vi "Launcher.vi"   [LabVIEW 2019]
uses:
  My First Actor.lvclass
  C:/Program Files (x86)/National Instruments/LabVIEW 2019/vi.lib/ActorFramework/Actor/Actor.lvclass
  My First Actor Messages/PopUp Msg/PopUp Msg.lvclass/PopUp Msg.ctl
  <vilib>/ActorFramework/Message Enqueuer/Message Enqueuer.lvclass/Message Enqueuer.ctl
  My First Actor Messages/PopUp2 Msg/PopUp2 Msg.lvclass/PopUp2 Msg.ctl
  <vilib>/ActorFramework/Message Enqueuer/Enqueue.vi
  My First Actor Messages/PopUp Msg/PopUp Msg.lvclass
  C:/Program Files (x86)/National Instruments/LabVIEW 2019/vi.lib/ActorFramework/Message/Message.lvclass
  My First Actor Messages/PopUp2 Msg/PopUp2 Msg.lvclass
  <vilib>/ActorFramework/Stop Msg/Stop Msg.lvclass
  <vilib>/ActorFramework/Message Priority Queue/Priority Enqueue.vi
  <vilib>/ActorFramework/Actor/Actor.lvclass
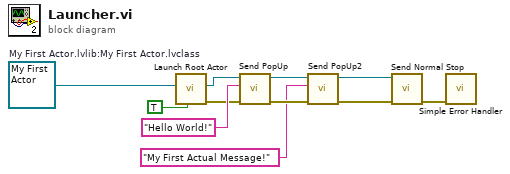
[diagram p0: block diagram]
diagram:
  w11 = refnum<class "My First Actor.lvclass"> refnum  # My First Actor.lvlib:My First Actor.lvclass
  n1 = call <vilib>:"Launch Root Actor.vi"("Open Actor Core front panel? (F)"=TRUE, "Actor"=w11) -> ("error out"=w8:errorcluster, "Actor's Enqueuer"=w10:refnum<class "Message Enqueuer.lvclass">)  [unwired: 8 in]
  n2 = call "Send PopUp.vi"("error in (no error)"=w8, "String"="Hello World!", "Message Enqueuer"=w10) -> ("error out"=w5:errorcluster, "Message Enqueuer out"=w7:refnum<class "Message Enqueuer.lvclass">)  [unwired: 7 in]
  n3 = call "Send PopUp2.vi"("error in (no error)"=w5, "message"="My First Actual Message!" ("String"), "Message Enqueuer"=w7) -> ("error out"=w4:errorcluster, "Message Enqueuer out"=w6:refnum<class "Message Enqueuer.lvclass">)  [unwired: 7 in]
  n4 = call <vilib>:"Send Normal Stop.vi"("error in (no error)"=w4, "Message Enqueuer"=w6) -> ("error out"=w3:errorcluster)  [unwired: 9 in]
  n5 = call <vilib>:"Simple Error Handler.vi"("error in (no error)"=w3) -> ()  [unwired: 4 in, 5 out]
